vi "Point&Path@Circle2DPath__Parameter.vi"(1 "ParamterIn":string) -> (0 "ParamterOut":string)   [LabVIEW 2020]
panel:
  in  "Number":string(combo)
  in  "End":string(combo)
  in  "Start":string(combo)
  in  "PointName":string(combo)
  in  "Confirm":bool
  # "Point&Path@Circle2DPath $Point,$Start Angle,$End Angle,$Number\n$Point.X= X of Circle\n$Point.Y= Y of Circle\n$Point.H= Radius of Circle"
  # "~"
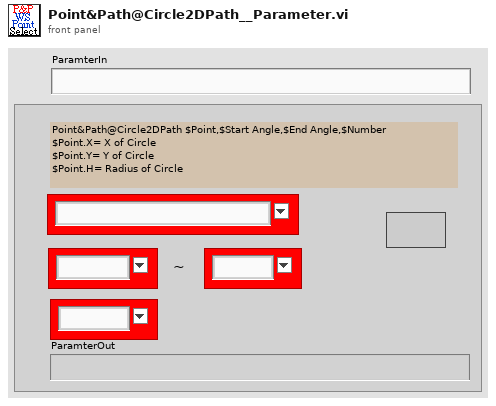
[diagram p1: front panel]
types:
  T1 = enum16{"Get", "UpdatePointS", "Init", "UpdateIndex", "GetCurrent&Index+1", "GetWithIndex", "ChkLast", "GetCurrent"}
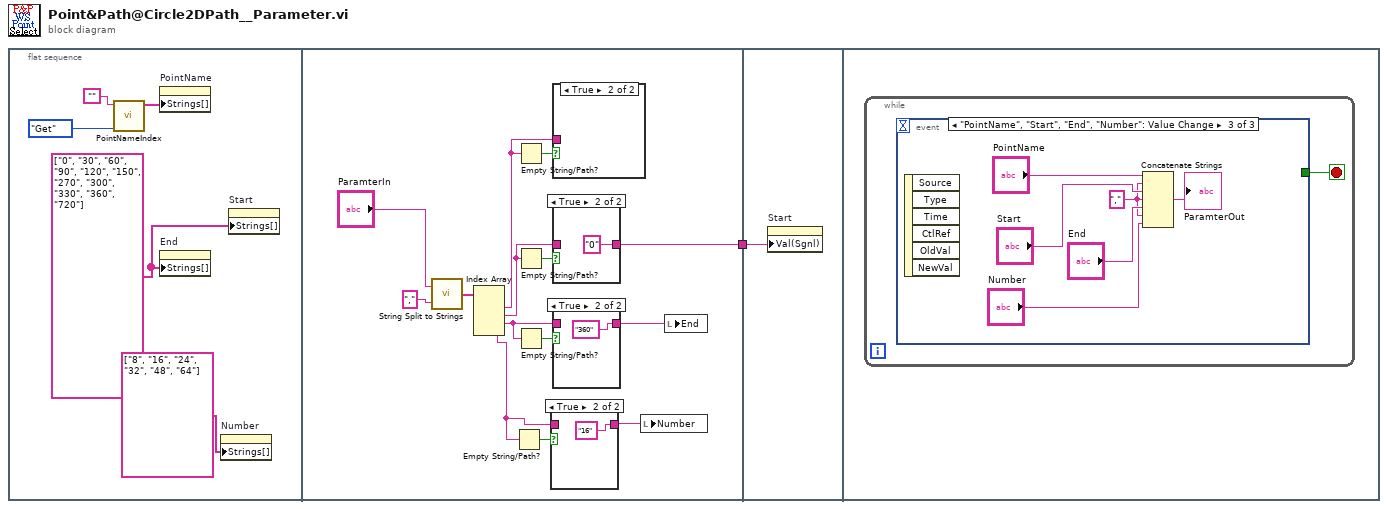
[diagram p0: block diagram]
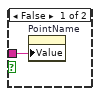
[diagram p5: hidden frame]
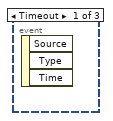
[diagram p6: hidden frame]
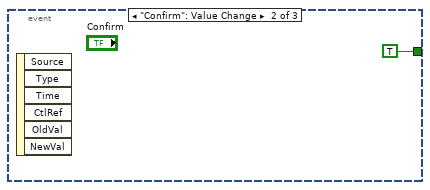
[diagram p7: hidden frame]
diagram:
  n1 = flat-sequence {
    tunnel: [w18] -> w1
    tunnel: w1 -> [w28]
    frame #0 {
      w3 = string[] ["0", "30", "60", "90", "120", "150", "270", "300", "330", "360", "720"] ("Strings []")
      n2 = call "PointNameIndex.vi"("OP"=T1."Get", "PointName"="") -> ("PointNameList"=w4:string[])  [unwired: 4 in, 5 out]
      n3 = property on="PointName" class="CmbBox"("Strings[]"=w4) -> ()  [unwired: 2 in, 2 out]
      n4 = property on="End" class="CmbBox"("Strings[]"=w3) -> ()  [unwired: 2 in, 2 out]
      n5 = property on="Number" class="CmbBox"("Strings[]"=string[] ["8", "16", "24", "32", "48", "64"] ("Strings []")) -> ()  [unwired: 2 in, 2 out]
      n6 = property on="Start" class="CmbBox"("Strings[]"=w3) -> ()  [unwired: 2 in, 2 out]
    }
    frame #1 {
      n7 = call "String Split to Strings.vi"("search string/char (-)"=",", "String"="ParamterIn") -> ("Array"=w16:string[])
      n8 = Index Array(array=w16) -> (element #1=w15:string, element #2=w14:string, element #3=w12:string, element #4=w8:string)  [unwired: 4 in]
      n9 = Empty String/Path?(string/path=w8) -> (empty?=w9:bool)
      n10 = Empty String/Path?(string/path=w15) -> (empty?=w20:bool)
      n11 = Empty String/Path?(string/path=w14) -> (empty?=w19:bool)
      n12 = Empty String/Path?(string/path=w12) -> (empty?=w13:bool)
      n13 = case shown="True" w9 {
        tunnel: [w21 "16" ("ParamterIn")] -> w7
        tunnel: w8 -> [w21 _]
        frame False {
        }
        frame True {
        }
      }
      n14 = case shown="True" w20 {
        tunnel: w15 -> [w27 _]
        frame False {
          n15 = property on="PointName" class="CmbBox"("Value"=w27) -> ()  [unwired: 2 in, 2 out]
        }
        frame True {
        }
      }
      n16 = case shown="True" w19 {
        tunnel: [w25 "0" ("ParamterIn")] -> w18
        tunnel: w14 -> [w25 _]
        frame False {
        }
        frame True {
        }
      }
      n17 = case shown="True" w13 {
        tunnel: [w23 "360" ("ParamterIn")] -> w11
        tunnel: w12 -> [w23 _]
        frame False {
        }
        frame True {
        }
      }
      n18 = local write "Number"(w7) -> ()
      n19 = local write "End"(w11) -> ()
    }
    frame #2 {
      n20 = property on="Start" class="CmbBox"("Val(Sgnl)"=w28) -> ()  [unwired: 2 in, 2 out]
    }
    frame #3 {
      n21 = while {
        stop <- w29 stop-if-true
        n22 = event shown="[2] \"PointName\", \"Start\", \"End\", \"Number\": Value Change" {
          selector: _ -> [_ _ _]
          dyn-events: _ -> [_ _ _]
          timeout: _ -> [_ _ _]
          tunnel: [_ TRUE _] -> w29
          event Timeout {
            n23 = event-data() -> ()  [unwired: 1 in, 3 out]
          }
          event "Confirm": Value Change {
            n24 = event-data() -> ()  [unwired: 1 in, 6 out]
          }
          event "PointName", "Start", "End", "Number": Value Change {
            w32 = ","
            n25 = event-data() -> ()  [unwired: 1 in, 6 out]
            n26 = Concatenate Strings("PointName", w32, "Start", w32, "End", w32, "Number") -> (→"ParamterOut":string)
          }
        }
      }
    }
  }
